vi "Increment.vi"(8 "error in (no error)":errorcluster, 10 "Numeric":dbl, 11 "TestActor in":refnum<class "TestActor.lvclass">) -> (0 "error out":errorcluster, 3 "TestActor out":refnum<class "TestActor.lvclass">)   [LabVIEW 2020, in "Messaging Tests.lvlib" / "TestActor.lvclass"]
uses:
  TestActor.lvclass
  TestActor.lvclass/TestActor.ctl
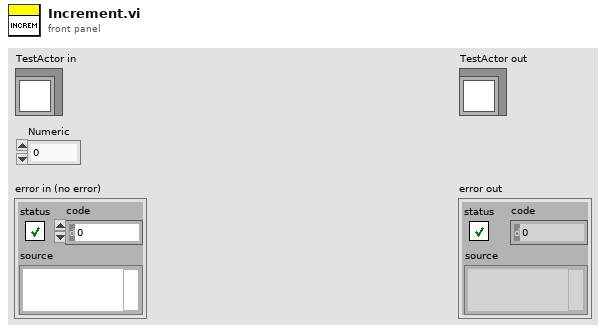
[diagram p1: front panel]
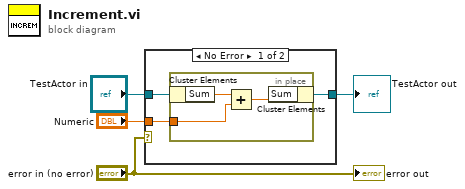
[diagram p0: block diagram]
diagram:
  n1 = case shown="No Error" "error in (no error)" {
    tunnel: [w6 w11] -> w2
    tunnel: "TestActor in" -> [w7 w11]
    tunnel: "Numeric" -> [w5 _]
    frame No Error {
      n2 = in-place {
        in-place-border: w5 -> [w9]
        n3 = in-place-cluster #1(w7) -> ("Sum"=w10:dbl)
        n4 = Add(x=w10, y=w9) -> (x+y=w8:dbl)
        n5 = in-place-cluster #1("Sum"=w8) -> (w6:refnum<class "TestActor.lvclass">)
      }
    }
    frame Error {
    }
  }
  "TestActor out" <- w2
  "error out" <- "error in (no error)"
